vi "Read Channel Active.vi"(8 "error in":errorcluster, 11 "Output Channels in":refnum<class "Output Channels.lvclass">) -> (0 "error out":errorcluster, 2 "Channel Active":bool, 3 "Output Channels out":refnum<class "Output Channels.lvclass">)   [LabVIEW 2020, in "Plugin.lvlib" / "Output Channels.lvclass"]
doc: "Reads Channel Active."
uses:
  Output Channels.lvclass
  Output Channels.lvclass/Output Channels.ctl
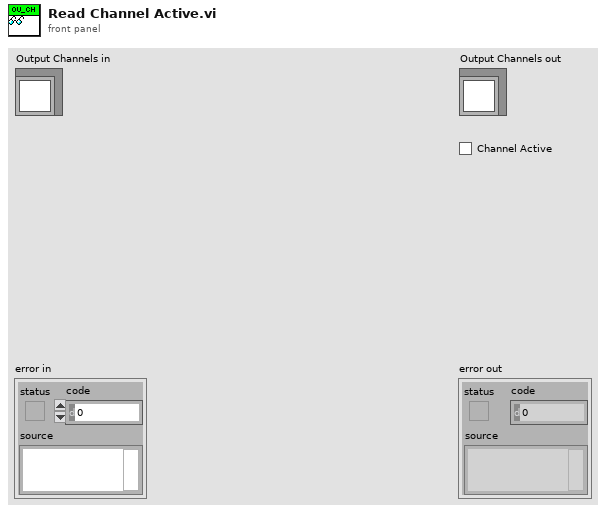
[diagram p1: front panel]
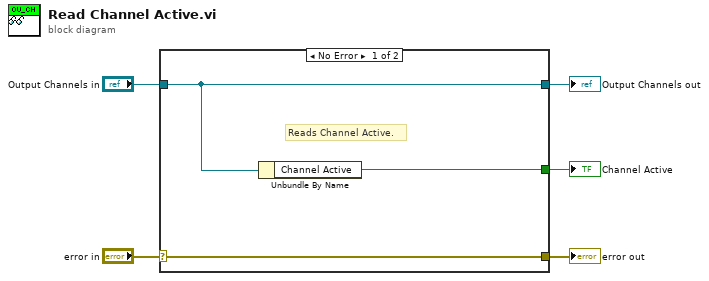
[diagram p0: block diagram]
diagram:
  n1 = case shown="No Error" "error in" {
    selector: "error in" -> [w8 w9]
    tunnel: [w8 w9] -> w4
    tunnel: [w7 w10] -> w2
    tunnel: "Output Channels in" -> [w7 w10]
    tunnel: [w6 _] -> w1
    frame No Error {
      # "Reads Channel Active."
      n2 = Unbundle By Name(w7) -> ("Channel Active"=w6:bool)
    }
    frame Error {
    }
  }
  "error out" <- w4
  "Output Channels out" <- w2
  "Channel Active" <- w1
